vi "globalSetUp.vi"(8 "error in":errorcluster, 11 "Single Core Simple Loopback in":refnum<class "Single Core Simple Loopback.lvclass">) -> (0 "error out":errorcluster, 3 "Single Core Simple Loopback out":refnum<class "Single Core Simple Loopback.lvclass">)   [LabVIEW 2020, in "Single Core Simple Loopback.lvclass"]
uses:
  Single Core Simple Loopback.lvclass
  niveristand-custom-device-testing-tools/VeriStandTestUtilities/VeriStandTestUtilities.lvlib
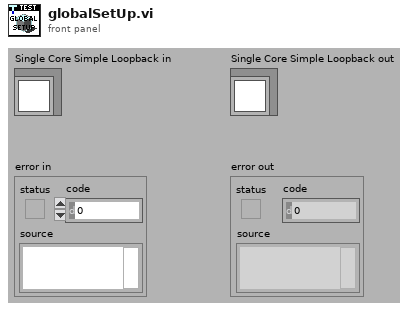
[diagram p1: front panel]
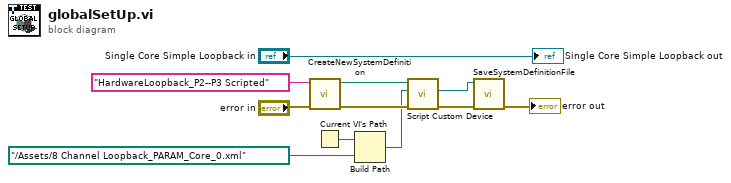
[diagram p0: block diagram]
diagram:
  n1 = call "CreateNewSystemDefinition.vi"("error in"="error in", "System Definition Name"="HardwareLoopback_P2--P3 Scripted" ("Channel")) -> ("error out"=w5:errorcluster, "System Definition Path"=w4:path)  [unwired: 8 in]
  n2 = Current VI's Path() -> (path=w11:path)
  n3 = Build Path(base path=w11, name or relative path=path "../Assets/8 Channel Loopback_PARAM_Core_0.xml" ("Hardware File Path")) -> (appended path=w1:path)
  n4 = call "Script Custom Device.vi"("error in"=w5, "Parameter File Path"=w1, "System Definition File Path In"=w4) -> ("error out"=w9:errorcluster, "System Definition Reference"=w2:refnum<k24>)  [unwired: 5 in, 2 out]
  n5 = call "SaveSystemDefinitionFile.vi"("error in (no error)"=w9, "System Definition Reference in"=w2) -> ("error out"=→"error out":errorcluster)  [unwired: 8 in, 1 out]
  "Single Core Simple Loopback out" <- "Single Core Simple Loopback in"
